vi "RAMP SPEED.vi"(8 "error in (no error)":errorcluster, 11 "main ref":T1) -> (0 "error out":errorcluster)   [LabVIEW 2025]
uses:
  controls/LAB-IQ UI Data.ctl
  SWAY vi's/Sway Write enum.ctl
  <vilib>/Analysis/1siggen.llb/Ramp Pattern by Samples.vi
  <vilib>/Analysis/NI_AALBase.lvlib
  HEAVE vi's/Heave Write enum.ctl
panel:
  out "Initial Rpm":dbl
  out "Wait Time":dbl
  out "Total Steps":dbl
  out "Speed":dbl
  out "Ramp Pattern":dbl[](array[numeric])
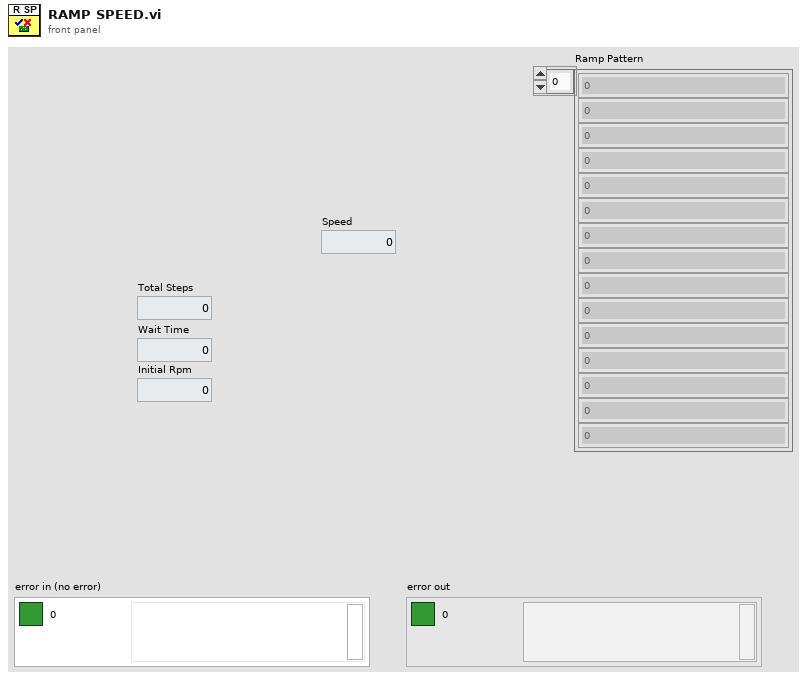
[diagram p1: front panel]
types:
  T1 = typedef "LAB-IQ UI Data.ctl" = cluster{"Main Home Screen":cluster{"GUI":refnum<vi>, "Platform Settings":refnum<vi>, "Configure":refnum<vi>, "Home":refnum<vi>, "EXIT":refnum<vi>, "service 2":refnum<vi>, "MainPage":refnum<vi>, "Analysis":refnum<vi>}, "Platform Settings":cluster{"mm/s  Surge":refnum<vi>, "Update Surge Speed":refnum<vi>, "Drive Error":refnum<vi>, "Disable Axis Jog Soft Limits":refnum<vi>, "mm/s  Sway":refnum<vi>, "Sway and Surge COM Status":refnum<vi>, "Heave COM Status":refnum<vi>, "Enable Platform":refnum<vi>, "Surge Forward Main":refnum<vi>, "Sway Right Main":refnum<vi>, "Sway Left Main":refnum<vi>, "Heave Down Main":refnum<vi>, "Heave Up main":refnum<vi>, "Update Sway Speed":refnum<vi>, "Update Heave Speed":refnum<vi>, "mm/s Heave":refnum<vi>, "mm/sec":refnum<vi>, "mm":refnum<vi>, "Surge Backward Main":refnum<vi>}, "Analysis Screen":cluster{"Analysis Home":refnum<vi>, "Surface Analysis":refnum<vi>, "Imaging":refnum<vi>, "Image Analysis":refnum<vi>, "Post Analysis":refnum<vi>}, "Config Screen":cluster{"Select Load Head":refnum<vi>, "Notes :":refnum<vi>, "FILE":refnum<vi>, "Sample ID :":refnum<vi>, "Operator ID :":refnum<vi>, "Operator Name :":refnum<vi>, "Auto":refnum<vi>}, "Motion Module":cluster{"zNL":refnum<vi>, "NL disp":refnum<vi>, "Rotary Tab":refnum<vi>, "Motion Direction:  3":refnum<vi>, "E.Velocity 2":refnum<vi>, "e.v/ssr 2":refnum<vi>, "Enter Fixed E.Velocity 2":refnum<vi>, "Enter Final SRR 2":refnum<vi>, "Enter initial SRR 2":refnum<vi>, "Enter Fixed SRR 2":refnum<vi>, "Enter the Final E.Velocity (m/s) 2":refnum<vi>, "Enter initial E.Velocity (m/s) 2":refnum<vi>, "Final Speed (RPM) 3":refnum<vi>, "Initial Speed (RPM) 2":refnum<vi>, "Enter the Final Velocity (m/s) 3":refnum<vi>, "Enter initial Velocity (m/s)  3":refnum<vi>, "Ramp Up 2":refnum<vi>, "TEST SELECTION":refnum<vi>, "SPEED SELECTION : ":refnum<vi>, "Angular Oscillation Set":refnum<vi>, "Traction":refnum<vi>, "Step Speed":refnum<vi>, "StepTable For Load-Speed":refnum<vi>, "StepTable For Speed":refnum<vi>, "Surge Forward MM":refnum<vi>, "Surge Backward MM":refnum<vi>, "M3 Image":refnum<vi>, "String 39":refnum<vi>, "Sway Left MM":refnum<vi>, "Sway Right MM":refnum<vi>, "Disable Axis Jog Soft Limits":refnum<vi>, "mm":refnum<vi>, "Heave Down MM":refnum<vi>, "Heave Up MM":refnum<vi>, "Wear Track Diameter (mm)":refnum<vi>, "Set WTD":refnum<vi>, "HomeScratch":refnum<vi>, "HomeRot":refnum<vi>, "PlaceModule":refnum<vi>, "Enter the Angle (Deg)":refnum<vi>, "Enter the Frequency (Hz)":refnum<vi>, "Motion Mode:":refnum<vi>, "LR Sway":refnum<vi>, "Rot Hor":refnum<vi>, "Scratch":refnum<vi>, "LR Cam":refnum<vi>, "MMBack":refnum<vi>, "MMNext":refnum<vi>, "Rot Ver":refnum<vi>, "Rotary Module Selection":refnum<vi>, "calculate rotary":refnum<vi>, "SPEED SELECTION : rotary":refnum<vi>, "Import 2":refnum<vi>, "Save 2":refnum<vi>, "File Path :  2":refnum<vi>, "String 45":refnum<vi>, "StepTable For Speed 3":refnum<vi>, "Enter the Speed(mm/sec)":refnum<vi>, "Enter the Speed(RPM)":refnum<vi>, "Enter Scratch Speed (mm/s):":refnum<vi>, "SwaySpeed Set":refnum<vi>, "Scartch Offset":refnum<vi>, "Motion type:":refnum<vi>, "HomeScratch 2":refnum<vi>, "Enter Scratch length (mm):":refnum<vi>, "Wear Track Diameter":refnum<vi>, "Rotary Speed Exced":refnum<vi>, "Scratch Mode":refnum<vi>, "No of Scratch":refnum<vi>}, "Environmental control":cluster{"Humidity  Status  3":refnum<vi>, "Low Temp  Status  2":refnum<vi>, "TK4 status 2":refnum<vi>, "Stage Temperature":refnum<vi>, "Sample Temperature":refnum<vi>, "Humidity (Amb)":refnum<vi>, "Clear List":refnum<vi>, "Add to list":refnum<vi>, "Wear":refnum<vi>, "Vibration":refnum<vi>, "Humidity (Chamber)":refnum<vi>, "Temperature (Chamber)":refnum<vi>, "ECR ":refnum<vi>, "Temperature (Amb)":refnum<vi>, "Microphone":refnum<vi>, "Acoustic Emission 3":refnum<vi>, "SNext":refnum<vi>, "APBack":refnum<vi>, "Enter the Temperature (°C):":refnum<vi>, "Enter the Stage \nTemperature (°C):":refnum<vi>, "Enter the Humidity (%Rh):":refnum<vi>, "Low Temp":refnum<vi>, "High Temp":refnum<vi>, "Humidity":refnum<vi>, "Sensors Picked":refnum<vi>}, "About Screen":cluster{"Password":refnum<vi>, "Home Service":refnum<vi>, "Advanced Setting":refnum<vi>, "About Tab":refnum<vi>, "ECR Port:":refnum<vi>, "Ramp Port:":refnum<vi>, "Installation/Replacement completed":refnum<vi>, "Loahead":refnum<vi>, "Heave and Surge COM Port:":refnum<vi>, "Sway COM Port:":refnum<vi>, "Temp Modbus:":refnum<vi>, "Humidity Port:":refnum<vi>, "Edit Gain Constants":refnum<vi>, "Save Gain Constants":refnum<vi>}, "Main Screen":cluster{"Main Screen Tab":refnum<vi>, "Angle and Frequency":refnum<vi>, "Stroke (mm)":refnum<vi>, "Angle (Deg)":refnum<vi>, "Main Speed Tab":refnum<vi>, "MTM MOTOR DISPLAY":refnum<vi>, "Disc Speed (m/sec)":refnum<vi>, "Ball Speed (m/sec)":refnum<vi>, "Disc Speed (RPM)":refnum<vi>, "Ball Speed (RPM)":refnum<vi>, "SPEED TAB":refnum<vi>, "Speed (m/sec)":refnum<vi>, "Set Speed (m/sec)":refnum<vi>, "Speed (RPM)":refnum<vi>, "Set Speed":refnum<vi>, "Time Tab":refnum<vi>, "Time ( HH:MM:SS ) 2":refnum<vi>, "Test Duration":refnum<vi>, "Test Duration 4":refnum<vi>, "TEST CYCLE":refnum<vi>, "TOTAL CYCLES":refnum<vi>, "Set Load (N)":refnum<vi>, "Temp Tabs":refnum<vi>, "Heater":refnum<vi>, "TK4 status":refnum<vi>, "ChamberTemp":refnum<vi>, "SetTmp":refnum<vi>, "Controller  Status":refnum<vi>, "ChamberTemp 2":refnum<vi>, "SetTmp 2":refnum<vi>, "Controller  Status 2":refnum<vi>, "ChamberTemp 3":refnum<vi>, "SetTmp 3":refnum<vi>, "Cooling":refnum<vi>, "Load Communication":refnum<vi>, "Ambient \nTemperature":refnum<vi>, "HumCOMStatus":refnum<vi>, "Ambient\n Humidity":refnum<vi>, "Freq (Hz)":refnum<vi>, "Load En":refnum<vi>, "NLt":refnum<vi>, "zNL 2":refnum<vi>, "Humidity On":refnum<vi>, "humidity disp":refnum<vi>, "Set Humidity":refnum<vi>, "NL disp 2":refnum<vi>, "Humidity On 2":refnum<vi>, "humidity disp 2":refnum<vi>, "Set Humidity 2":refnum<vi>, "NL disp 3":refnum<vi>, "AppLoadSeq scratch":refnum<vi>, "Stop Scratch":refnum<vi>, "ClrLog":refnum<vi>, "Trip Log":refnum<vi>, "STOP":refnum<vi>, "Start Test":refnum<vi>, "Test status":refnum<vi>, "AR Led":refnum<vi>, "Data":refnum<vi>, "Health":refnum<vi>, "Sway COM Status":refnum<vi>, "Heave COM Status":refnum<vi>, "Grp Tab":refnum<vi>, "Sub Graph":refnum<vi>, "SD (mm)":refnum<vi>, "Siliding distance Reset Graph":refnum<vi>, "SDGp":refnum<vi>, "Humidity Reset Graph":refnum<vi>, "HumrGp":refnum<vi>, "Acoustic Emission (mV)":refnum<vi>, "Aqucostic Reset Graph":refnum<vi>, "gACQUOS":refnum<vi>, "ECR RESET":refnum<vi>, "ECR":refnum<vi>, "Temperature Reset":refnum<vi>, "Acoustic Emission (mV) 2":refnum<vi>, "Aqucostic Reset Graph 2":refnum<vi>, "gACQUOS 2":refnum<vi>, "ECR RESET 2":refnum<vi>, "ECR 2":refnum<vi>, "Temperature Reset 2":refnum<vi>, "Temperature (deg c)":refnum<vi>, "Speed Reset Graph":refnum<vi>, "Speed Tab":refnum<vi>, "MTM DISC  SPEED":refnum<vi>, "MTM BALL SPEED":refnum<vi>, "speed mm/sec":refnum<vi>, "Hymidity":refnum<vi>, "Humidity Disable trip":refnum<vi>, "CoF Trip  2":refnum<vi>, "Depth Trip":refnum<vi>, "Weart Deapth":refnum<vi>, "Depth Reset Graph":refnum<vi>, "Weart":refnum<vi>, "Depthz":refnum<vi>, "Depth (µm)":refnum<vi>, "WearGp":refnum<vi>, "NL Trip 2":refnum<vi>, "Load pid":refnum<vi>, "Load Disable Trip":refnum<vi>, "Load Reset Graph":refnum<vi>, "NL Display 4":refnum<vi>, "Main Chart 3":refnum<vi>, "BACK":refnum<vi>, "Depth Trip 2":refnum<vi>, "COF TRIP ":refnum<vi>, "Friction Force (N)":refnum<vi>, "FF Reset Graph":refnum<vi>, "FF Disable Trip":refnum<vi>, "FF TRIP":refnum<vi>, "COF Disable Trip":refnum<vi>, "COF Reset Graph":refnum<vi>, "Start Test Temp":refnum<vi>, "zFF":refnum<vi>, "Friction Force (N) Graph":refnum<vi>, "Coefficient of Friction":refnum<vi>, "Scratch Start Test":refnum<vi>, "FF Tab":refnum<vi>, "Cyclic Friction Force (N)":refnum<vi>, "CZ FF":refnum<vi>, "Cyclic Friction Force (N) Graph":refnum<vi>, "Cyclic Coefficient of Friction":refnum<vi>, "Cyclic FF TRIP":refnum<vi>, "Cyclic FF Disable Trip":refnum<vi>, "cyclic COF Disable Trip":refnum<vi>, "cyclic COF TRIP":refnum<vi>, "cyclic COF Reset Graph":refnum<vi>, "Cyclic FF Reset Graph":refnum<vi>, "Test Trip":refnum<vi>, "Multi Scratch Pass":refnum<vi>, "Scratch Start Recording":refnum<vi>}, "Loading":cluster{"Indentation":refnum<vi>, "Reference Sample":refnum<vi>, "Load Cell Communication Slide":refnum<vi>, "com 3":refnum<vi>, "com":refnum<vi>, "DecaForce COM Status":refnum<vi>, "Update":refnum<vi>, "Clear 3":refnum<vi>, "seq":refnum<vi>, "Stribeck table":refnum<vi>, "Stribeck Table  For loading":refnum<vi>, "Loading Mode":refnum<vi>, "Enter the Final Load (N)":refnum<vi>, "Enter the CoF Trip":refnum<vi>, "Enter the Friction Force Trip":refnum<vi>, "Enter the Normal load Trip":refnum<vi>, "Enter the Load  (N)":refnum<vi>, "KiloForce":refnum<vi>, "DecaForce ":refnum<vi>, "MicroForce":refnum<vi>, "LHBack":refnum<vi>, "LHNext":refnum<vi>, "Enter the Loading Rate (N/min)":refnum<vi>, "Message":refnum<vi>, "Warning 2":refnum<vi>, "SSP 0.75":refnum<vi>, "SSP 0.5":refnum<vi>, "SSP 0.3":refnum<vi>, "Warning":refnum<vi>, "gui GIF":refnum<vi>, "Communication is established":refnum<vi>, "AppLoad 4":refnum<vi>, "Multipoint":refnum<vi>, "Load Selection":refnum<vi>}, "PID":cluster{"Ramp MulFac":refnum<vi>, "pulses LoadDiffRamp(2..10)":refnum<vi>, "PulseControlRamp(diff<=3N)":refnum<vi>, "SetLoadDeadband(%) Load(0-10N)":refnum<vi>, "PID gains out delay (microForce)":refnum<vi>, "Ramp":refnum<vi>, "Gain 2":refnum<vi>, "pulses LoadDiff(2..10)":refnum<vi>, "pulses LoadDiff(11..50)":refnum<vi>, "PulseControl(diff<=3N)":refnum<vi>, "SetLoadDeadband(%)  2":refnum<vi>, "Dummy Run":refnum<vi>, "Vertical load (N)":refnum<vi>, "AutoTune":refnum<vi>, "Offset 3 ":refnum<vi>, "apply load":refnum<vi>, "Offset  3":refnum<vi>, "apply load 2":refnum<vi>, "Enter ByPass Load":refnum<vi>, "reinit 3":refnum<vi>, "output range delay":refnum<vi>, "PID gains out delay":refnum<vi>, "Bypass Load":refnum<vi>, "pulsesSent":refnum<vi>, "pulses ":refnum<vi>, "actpid":refnum<vi>, "gFF Rot":refnum<vi>, "pulses LoadDiff(21..1000)":refnum<vi>, "Delay":refnum<vi>, "deadband":refnum<vi>}, "Config Parameters":cluster{"Tab Control 3":refnum<vi>, "Tab Control 19":refnum<vi>, "SAMPLES":refnum<vi>, "Re-initilaize":refnum<vi>, "Filter ON/OFF":refnum<vi>, "TracHomeSurgeOffsetCounts 10MM":refnum<vi>, "TracHomeSwayOffsetCounts 10MM":refnum<vi>, "Acoustic Emission:":refnum<vi>, "Apply Filter (FF)":refnum<vi>, "Filter% 2":refnum<vi>, "Apply Filter (Load)":refnum<vi>, "Filter% ":refnum<vi>, "Sway distance (mm)":refnum<vi>, "Surge distance (mm)":refnum<vi>, "DataSavingLoopDelay(ms)":refnum<vi>, "SAVE 2":refnum<vi>, "Enter Distance":refnum<vi>, "Sway Counts:":refnum<vi>, "Distance (mm): 3":refnum<vi>, "Surge Counts:":refnum<vi>, "Distance (mm): 2":refnum<vi>, "Distance (mm):":refnum<vi>, "Heave Counts:":refnum<vi>, "LRMHomeSurgeOffsetCounts":refnum<vi>, "LRMHomeSwayOffsetCounts":refnum<vi>, "TracHomeSurgeOffsetCounts 20MM":refnum<vi>, "TracHomeSwayOffsetCounts 20MM":refnum<vi>, "RotHomeSwayOffsetCounts":refnum<vi>, "RotHomeSurgeOffsetCounts":refnum<vi>, "Heave distance":refnum<vi>, "Zmm":refnum<vi>, "Heave Pulses/mm":refnum<vi>, "Surge Pulses/mm":refnum<vi>, "Sway Pulses/mm":refnum<vi>, "Heave Pitch":refnum<vi>, "Surge Pitch":refnum<vi>, "Sway Pitch":refnum<vi>, "Heave PPR":refnum<vi>, "Surge PPR":refnum<vi>, "Sway PPR":refnum<vi>, "Tab Control 5":refnum<vi>, "Tab Control 14":refnum<vi>, "Tab Control 26":refnum<vi>, "AE":refnum<vi>, "Heave Loop Delay":refnum<vi>, "Heave PID Speed":refnum<vi>, "Surge Jog Speed":refnum<vi>, "Heave Jog Speed":refnum<vi>, "Sway Loop Delay":refnum<vi>, "Sway PID Speed":refnum<vi>, "Sway Jog Speed":refnum<vi>, "DEPTH TRIP VALUE":refnum<vi>, "LOAD TRIP VALUE":refnum<vi>, "DEPTH TRIP   ENABLE":refnum<vi>, "LOAD TRIP  ENABLE":refnum<vi>, "CYCLIC FF TRIP VALUE":refnum<vi>, "FF TRIP VALUE":refnum<vi>, "CYCLIC CoF TRIP VALUE":refnum<vi>, "COF TRIP VALUE":refnum<vi>, "CYCLIC COF TRIP  ENABLE":refnum<vi>, "CYCLIC FF TRIP  ENABLE":refnum<vi>, "FF TRIP  ENABLE":refnum<vi>, "COF TRIP  ENABLE":refnum<vi>}, "Loading Com Port":cluster{"ClearAll":refnum<vi>, "Mz(Nm)":refnum<vi>, "My(Nm)":refnum<vi>, "Mx(Nm)":refnum<vi>, "Save Dwell":refnum<vi>, "Mx ":refnum<vi>, "My ":refnum<vi>, "Mz":refnum<vi>, "Fx(N)":refnum<vi>, "Fy(N)":refnum<vi>, "Fz(N)":refnum<vi>, "ZeroAll":refnum<vi>, "Acq Delay (ms)":refnum<vi>, "Burst Delay (ms)":refnum<vi>, "model":refnum<vi>, "SN":refnum<vi>, "FFx(N)":refnum<vi>, "Sensor IP":refnum<vi>, "Port":refnum<vi>, "FFy(N)":refnum<vi>, "Load(N)":refnum<vi>, "delete Handle":refnum<vi>, "Create Handle":refnum<vi>, "ft_data":refnum<vi>, "ft_range":refnum<vi>, "ft_data 2":refnum<vi>, "stop 6":refnum<vi>, "running_flag":refnum<vi>, "ft_udp_handle":refnum<vi>, "get-data-return":refnum<vi>, "get-range-return":refnum<vi>, "zero-return":refnum<vi>, "filter-return":refnum<vi>, "initial-return":refnum<vi>, "deleteHandle-result":refnum<vi>, "Load Cell Temp":refnum<vi>}, "Heave AND Surge":cluster{"SURGE POSE":refnum<vi>, "error out Read":refnum<vi>, "HEAVE POSE":refnum<vi>, "State":refnum<vi>, "Homed":refnum<vi>, "Sequence ID":refnum<vi>, "error out Write":refnum<vi>, "faultCode":refnum<vi>, "Ack ID":refnum<vi>, "SPEED":refnum<vi>, "Distance":refnum<vi>, "Mode Command":refnum<vi>, "Heave and Surge Read":refnum<vi>, "Read Heave Temp":refnum<vi>, "Spare 15":refnum<vi>, "Spare 14":refnum<vi>, "Spare 13":refnum<vi>, "Spare 12":refnum<vi>, "Spare 11":refnum<vi>, "Spare 10":refnum<vi>, "Spare 9":refnum<vi>, "Spare 8":refnum<vi>, "Spare 7":refnum<vi>, "Spare 6":refnum<vi>, "Spare 5":refnum<vi>, "Spare 4":refnum<vi>, "Spare 2":refnum<vi>, "Spare 1":refnum<vi>, "Node Id":refnum<vi>, "Spare 3":refnum<vi>, "SPARE 4":refnum<vi>, "SPARE 3":refnum<vi>, "SPARE 2":refnum<vi>, "SPARE 1":refnum<vi>, "fwMajor":refnum<vi>, "fwMinor":refnum<vi>, "Manual Write":refnum<vi>, "Heave and Surge Write":refnum<vi>}, "New PID LOGIC":cluster{"Fine Tune Zone":refnum<vi>, "PID SDelay":refnum<vi>, "Max_pos_limit":refnum<vi>, "Min_pos_limit":refnum<vi>, "i_limit":refnum<vi>, "pct_scale":refnum<vi>, "Deadband":refnum<vi>, "Kd":refnum<vi>, "Ki":refnum<vi>, "Kp":refnum<vi>, "Current Position":refnum<vi>, "Set Load":refnum<vi>, "Current Load":refnum<vi>, "Pulse delta":refnum<vi>, "Init Step":refnum<vi>, "Max Step Linit":refnum<vi>}, "SWAY ":cluster{"fwMajor":refnum<vi>, "Homed":refnum<vi>, "Rotary POSE":refnum<vi>, "State":refnum<vi>, "SWAY POSE":refnum<vi>, "Ack ID":refnum<vi>, "faultCode":refnum<vi>, "Node Id":refnum<vi>, "fwMinor":refnum<vi>, "Spare 6":refnum<vi>, "Spare 5":refnum<vi>, "Spare 4":refnum<vi>, "Spare 3":refnum<vi>, "Spare 2":refnum<vi>, "Spare 1":refnum<vi>, "Spare 7":refnum<vi>, "SPARE  5":refnum<vi>, "error out Write  SWAY ":refnum<vi>, "error out Read SWAY ":refnum<vi>, "Manual Write SWAY ":refnum<vi>, "SWAY WRITE":refnum<vi>, "SPARE  4":refnum<vi>, "SPARE  3":refnum<vi>, "SPARE 2":refnum<vi>, "SPARE 1":refnum<vi>, "Spare 15":refnum<vi>, "Spare 14":refnum<vi>, "Spare 13":refnum<vi>, "Spare 12":refnum<vi>, "Spare 11":refnum<vi>, "Spare 9":refnum<vi>, "Spare 8":refnum<vi>, "SPEED":refnum<vi>, "Distance":refnum<vi>, "Mode Command":refnum<vi>, "Sequence ID":refnum<vi>, "SWAY READ":refnum<vi>, "Spare 10":refnum<vi>, "Read SWAY Temp":refnum<vi>}, "Analysis Screen":cluster{"Analysis Home":refnum<vi>, "Refresh 2":refnum<vi>, "MEAN 4":refnum<vi>, "SD 4":refnum<vi>, "VARIANCE 4":refnum<vi>, "MEAN  3":refnum<vi>, "SD  3":refnum<vi>, "VARIANCE  3":refnum<vi>, "MEAN 2":refnum<vi>, "SD  2":refnum<vi>, "VARIANCE 2":refnum<vi>, "MEAN":refnum<vi>, "SD":refnum<vi>, "VARIANCE":refnum<vi>, "File 4 Discription":refnum<vi>, "OPEN 4":refnum<vi>, "File Name 4":refnum<vi>, "OPEN 3":refnum<vi>, "File 3 Discription":refnum<vi>, "File Name 3":refnum<vi>, "Y-AXIS":refnum<vi>, "X-AXIS":refnum<vi>, "XY Graph":refnum<vi>, "File Name 2":refnum<vi>, "File Name 1":refnum<vi>, "OPEN 2":refnum<vi>, "OPEN 1":refnum<vi>, "File 1 Discription ":refnum<vi>, "File 2 Discription":refnum<vi>, "Export":refnum<vi>, "File Format":refnum<vi>}}
  T2 = enum32{"Setup", "Load Head", "Motion Module", "Environment", "Begin"}
  T3 = typedef "Sway Write enum.ctl" = enum16{"INIT", "WRITE", "CLOSE", "REINIT"}
  T4 = typedef "Heave Write enum.ctl" = enum16{"INIT", "WRITE", "CLOSE", "REINIT"}
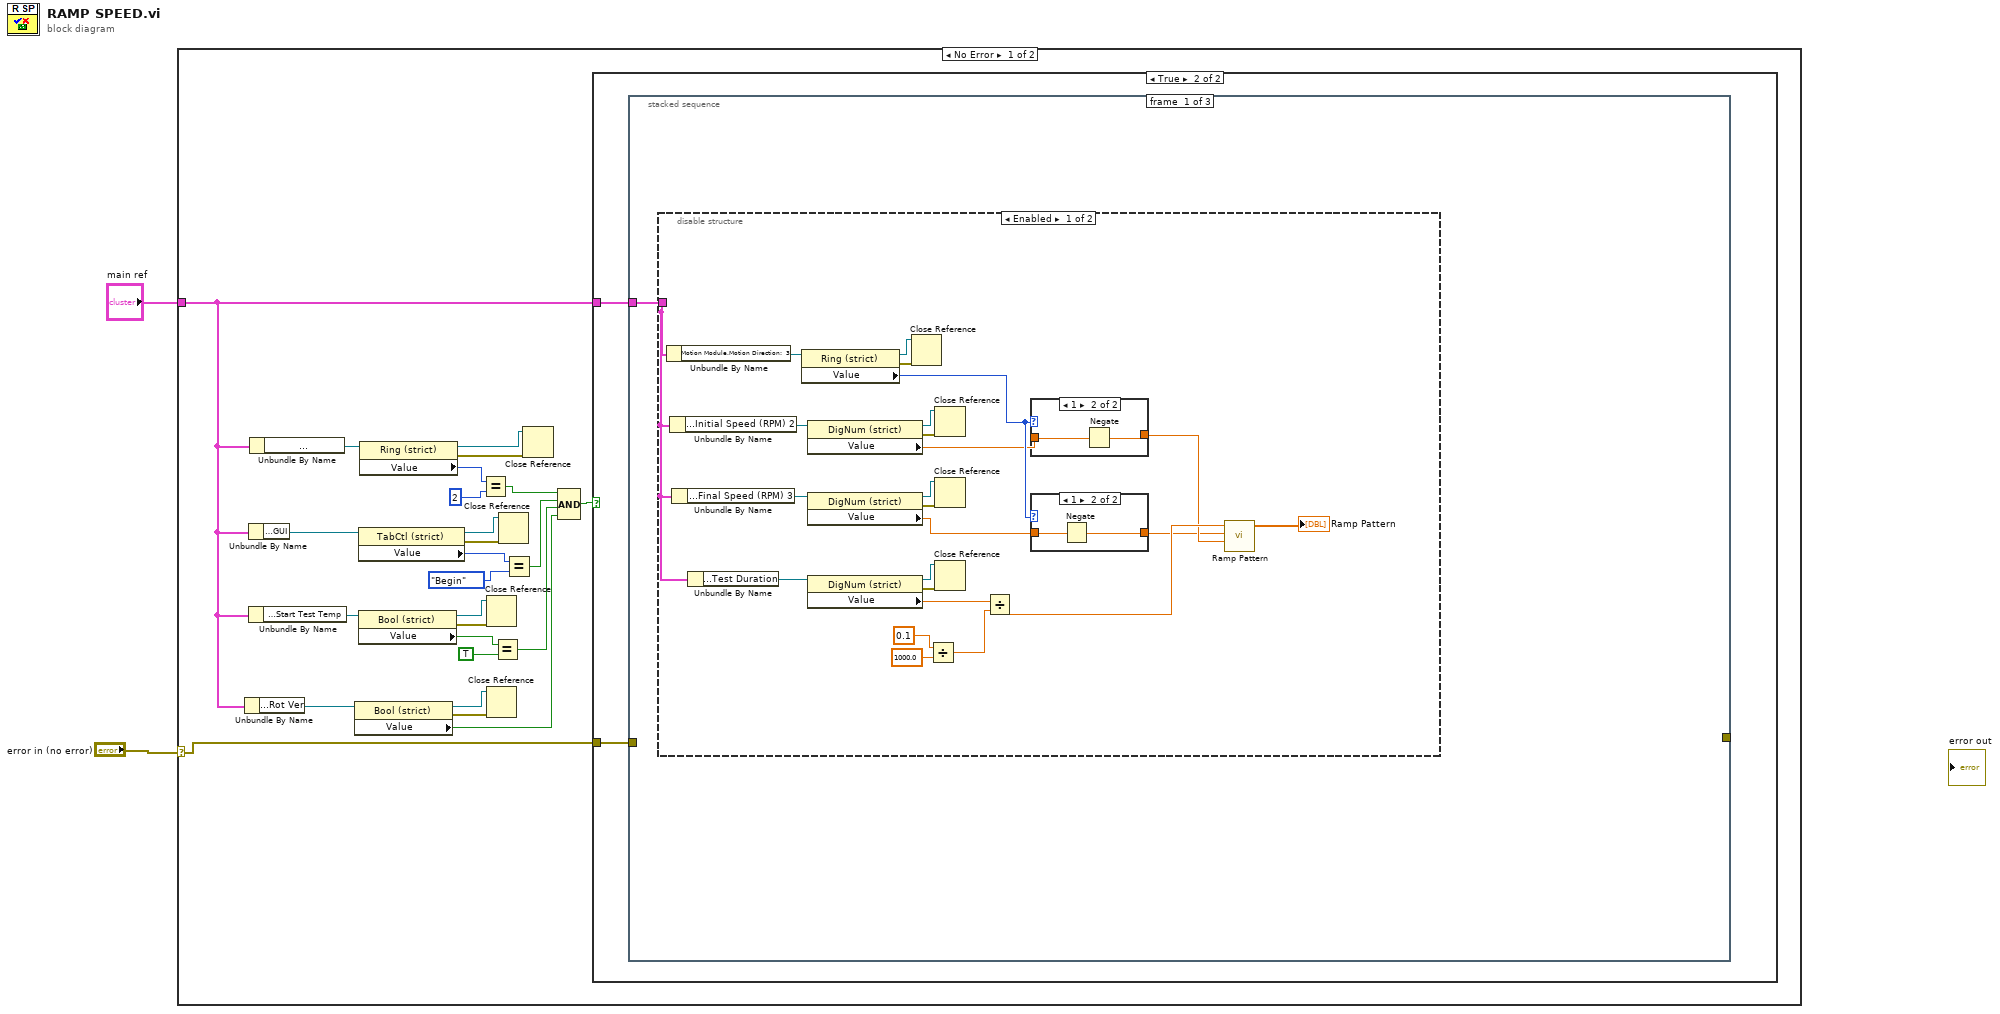
[diagram p0: block diagram]
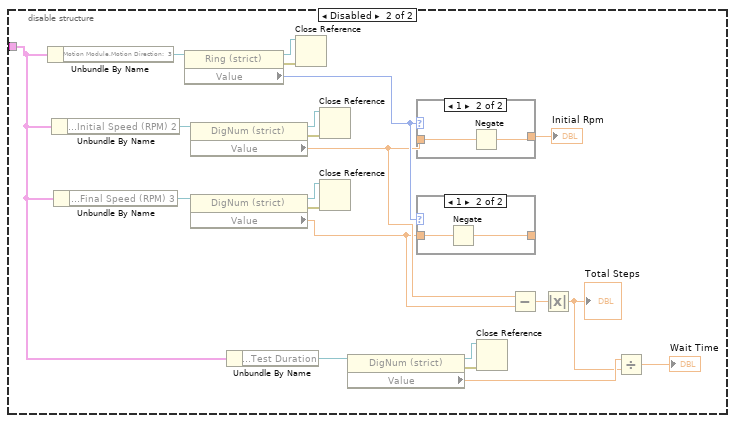
[diagram p5: hidden frame]
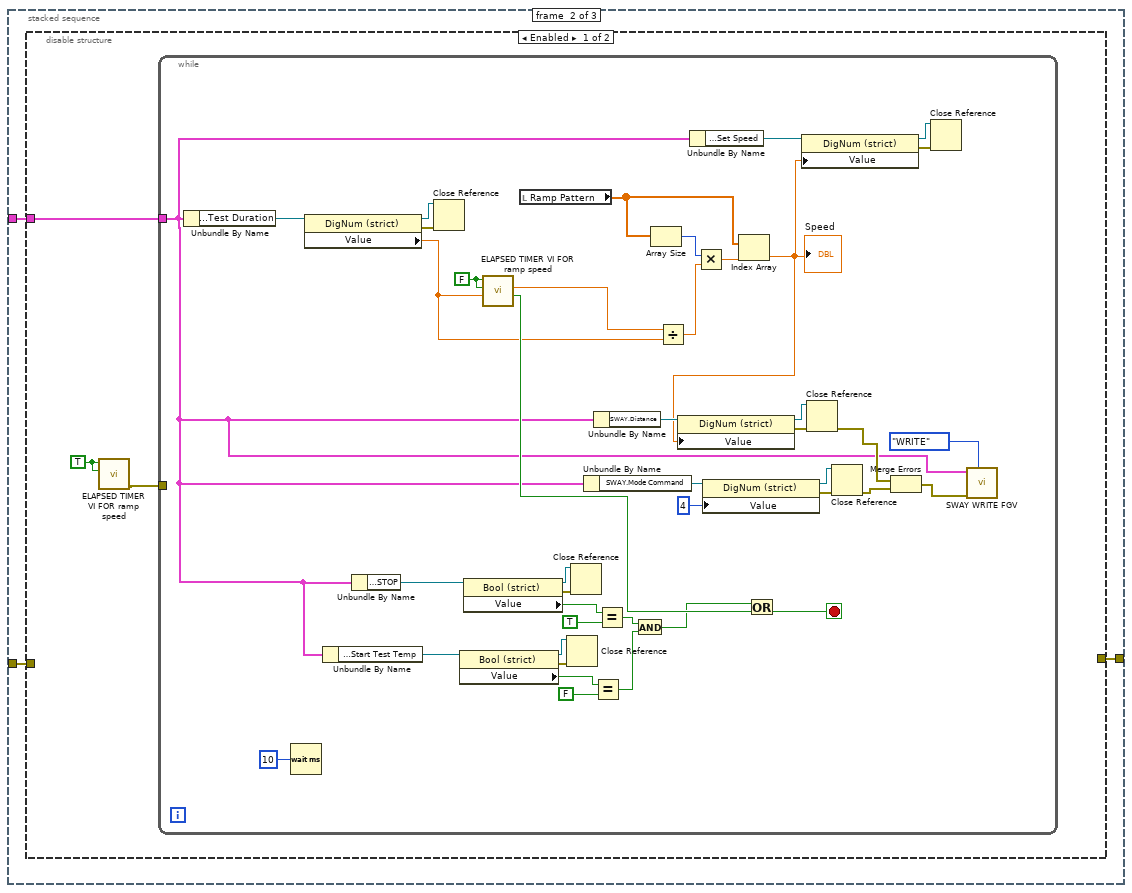
[diagram p8: hidden frame]
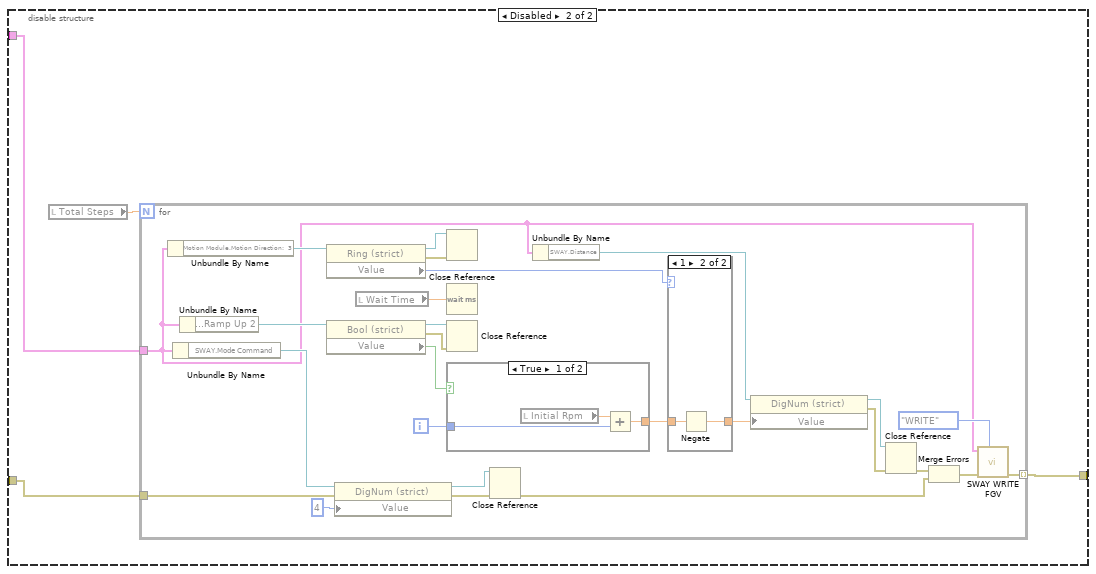
[diagram p9: hidden frame]
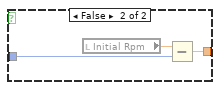
[diagram p10: hidden frame]
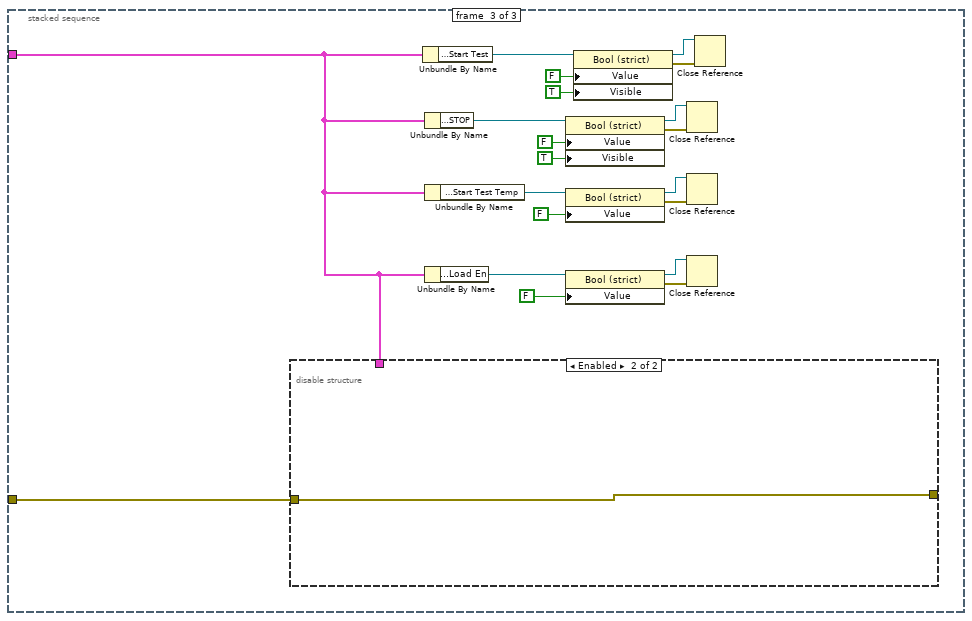
[diagram p12: hidden frame]
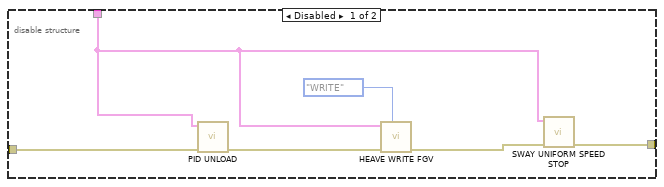
[diagram p13: hidden frame]
diagram:
  n1 = case shown="No Error" "error in (no error)" {
    selector: "error in (no error)" -> [w3 _]
    tunnel: "main ref" -> [w5 _]
    frame No Error {
      n2 = Unbundle By Name(w5) -> ("Motion Module.Rot Ver"=w9:refnum<vi>)
      n3 = Unbundle By Name(w5) -> ("Main Home Screen.GUI"=w19:refnum<vi>)
      n4 = Unbundle By Name(w5) -> ("Main Screen.Start Test Temp"=w14:refnum<vi>)
      n5 = Unbundle By Name(w5) -> ("Motion Module.Motion Mode:"=w27:refnum<vi>)
      n6 = property class="Bool (strict)"(reference=w9) -> (reference out=w6:refnum<vi>, error out=w8:errorcluster, "Value"=w7:bool)  [unwired: 1 in]
      n7 = property class="TabCtl (strict)"(reference=w19) -> (reference out=w21:refnum<vi>, error out=w20:errorcluster, "Value"=w18:T2)  [unwired: 1 in]
      n8 = property class="Bool (strict)"(reference=w14) -> (reference out=w12:refnum<vi>, error out=w13:errorcluster, "Value"=w15:bool)  [unwired: 1 in]
      n9 = property class="Ring (strict)"(reference=w27) -> (reference out=w25:refnum<vi>, error out=w26:errorcluster, "Value"=w24:u16)  [unwired: 1 in]
      n10 = Equal?(x=w24, y=u16 2 ("Value")) -> (x = y?=w22:bool)
      n11 = Close Reference(reference=w12, error in (no error)=w13) -> ()  [unwired: 1 out]
      n12 = Close Reference(reference=w6, error in (no error)=w8) -> ()  [unwired: 1 out]
      n13 = Equal?(x=w15, y=TRUE) -> (x = y?=w11:bool)
      n14 = Close Reference(reference=w21, error in (no error)=w20) -> ()  [unwired: 1 out]
      n15 = Equal?(x=w18, y=T2."Begin" ("Value")) -> (x = y?=w16:bool)
      n16 = Close Reference(reference=w25, error in (no error)=w26) -> ()  [unwired: 1 out]
      n17 = Compound Arithmetic op=AND(w22, w16, w11, w7) -> (w4:bool)
      n18 = case shown="True" w4 {
        tunnel: w5 -> [_ w29]
        tunnel: w3 -> [_ w28]
        frame False {
        }
        frame True {
          n19 = stacked-sequence {
            tunnel: w29 -> [w30 w90 w175]
            tunnel: w28 -> [_ w89 w176]
            tunnel: [_ w88 _] -> _
            frame #0 {
              n20 = disable-structure shown="Enabled" {
                disable-tunnel: w30 -> [w32 w68]
                frame Enabled {
                  n21 = Unbundle By Name(w32) -> ("Motion Module.Motion Direction:  3"=w47:refnum<vi>)
                  n22 = Unbundle By Name(w32) -> ("Motion Module.Initial Speed (RPM) 2"=w41:refnum<vi>)
                  n23 = Unbundle By Name(w32) -> ("Motion Module.Final Speed (RPM) 3"=w40:refnum<vi>)
                  n24 = Unbundle By Name(w32) -> ("Main Screen.Test Duration"=w33:refnum<vi>)
                  n25 = property class="Ring (strict)"(reference=w47) -> (reference out=w45:refnum<vi>, error out=w46:errorcluster, "Value"=w44:u16)  [unwired: 1 in]
                  n26 = property class="DigNum (strict)"(reference=w41) -> (reference out=w43:refnum<vi>, error out=w42:errorcluster, "Value"=w36:dbl)  [unwired: 1 in]
                  n27 = property class="DigNum (strict)"(reference=w40) -> (reference out=w38:refnum<vi>, error out=w39:errorcluster, "Value"=w37:dbl)  [unwired: 1 in]
                  n28 = property class="DigNum (strict)"(reference=w33) -> (reference out=w35:refnum<vi>, error out=w34:errorcluster, "Value"=w31:dbl)  [unwired: 1 in]
                  n29 = Close Reference(reference=w45, error in (no error)=w46) -> ()  [unwired: 1 out]
                  n30 = Divide(x=0.1 ("seconds to wait"), y=1000.0) -> (x/y=w54:dbl)
                  n31 = Close Reference(reference=w43, error in (no error)=w42) -> ()  [unwired: 1 out]
                  n32 = Close Reference(reference=w38, error in (no error)=w39) -> ()  [unwired: 1 out]
                  n33 = Close Reference(reference=w35, error in (no error)=w34) -> ()  [unwired: 1 out]
                  n34 = Divide(x=w31, y=w54) -> (x/y=w53:dbl)
                  n35 = case shown="1" w44 {
                    tunnel: w36 -> [w58 w60]
                    tunnel: [w58 w59] -> w52
                    frame 0, Default {
                    }
                    frame 1 {
                      n36 = Negate(x=w60) -> (-x=w59:dbl)
                    }
                  }
                  n37 = case shown="1" w44 {
                    tunnel: w37 -> [w55 w57]
                    tunnel: [w55 w56] -> w51
                    frame 0, Default {
                    }
                    frame 1 {
                      n38 = Negate(x=w57) -> (-x=w56:dbl)
                    }
                  }
                  n39 = call-poly <vilib>:"Ramp Pattern.vi"("start"=w52, "end"=w51, "samples"=w53) -> ("Ramp Pattern"=→"Ramp Pattern":dbl[])  [unwired: 7 in, 1 out]
                }
                frame Disabled {
                  n40 = Unbundle By Name(w68) -> ("Motion Module.Motion Direction:  3"=w81:refnum<vi>)
                  n41 = Unbundle By Name(w68) -> ("Motion Module.Initial Speed (RPM) 2"=w75:refnum<vi>)
                  n42 = Unbundle By Name(w68) -> ("Motion Module.Final Speed (RPM) 3"=w74:refnum<vi>)
                  n43 = property class="Ring (strict)"(reference=w81) -> (reference out=w79:refnum<vi>, error out=w80:errorcluster, "Value"=w78:u16)  [unwired: 1 in]
                  n44 = property class="DigNum (strict)"(reference=w75) -> (reference out=w77:refnum<vi>, error out=w76:errorcluster, "Value"=w67:dbl)  [unwired: 1 in]
                  n45 = property class="DigNum (strict)"(reference=w74) -> (reference out=w72:refnum<vi>, error out=w73:errorcluster, "Value"=w66:dbl)  [unwired: 1 in]
                  n46 = Unbundle By Name(w68) -> ("Main Screen.Test Duration"=w69:refnum<vi>)
                  n47 = Close Reference(reference=w79, error in (no error)=w80) -> ()  [unwired: 1 out]
                  n48 = Close Reference(reference=w77, error in (no error)=w76) -> ()  [unwired: 1 out]
                  n49 = Close Reference(reference=w72, error in (no error)=w73) -> ()  [unwired: 1 out]
                  n50 = property class="DigNum (strict)"(reference=w69) -> (reference out=w71:refnum<vi>, error out=w70:errorcluster, "Value"=w65:dbl)  [unwired: 1 in]
                  n51 = case shown="1" w78 {
                    tunnel: w67 -> [w85 w87]
                    tunnel: [w85 w86] -> w61
                    frame 0, Default {
                    }
                    frame 1 {
                      n52 = Negate(x=w87) -> (-x=w86:dbl)
                    }
                  }
                  "Initial Rpm" <- w61
                  n53 = case shown="1" w78 {
                    tunnel: w66 -> [w82 w84]
                    tunnel: [w82 w83] -> _
                    frame 0, Default {
                    }
                    frame 1 {
                      n54 = Negate(x=w84) -> (-x=w83:dbl)
                    }
                  }
                  n55 = Close Reference(reference=w71, error in (no error)=w70) -> ()  [unwired: 1 out]
                  n56 = Subtract(x=w67, y=w66) -> (x-y=w64:dbl)
                  n57 = Absolute Value(x=w64) -> (abs(x)=w63:dbl)
                  "Total Steps" <- w63
                  n58 = Divide(x=w65, y=w63) -> (x/y=→"Wait Time":dbl)
                }
              }
            }
            frame #1 {
              n59 = disable-structure shown="Enabled" {
                disable-tunnel: w90 -> [w91 w138]
                disable-tunnel: w89 -> [_ w137]
                disable-tunnel: [_ w136] -> w88
                frame Enabled {
                  w93 = TRUE ("PAUSE")
                  n60 = call "ELAPSED TIMER VI FOR ramp speed.vi"("RESET"=w93, "PAUSE"=w93) -> ("error out"=w92:errorcluster)  [unwired: 7 in, 2 out]
                  n61 = while {
                    tunnel: w92 -> [_]
                    tunnel: w91 -> [w94]
                    stop <- w111 stop-if-true
                    w134 = FALSE ("PAUSE")
                    n62 = Unbundle By Name(w94) -> ("Main Screen.Test Duration"=w126:refnum<vi>)
                    n63 = Wait (ms)(milliseconds to wait=u32 10) -> ()  [unwired: 1 out]
                    n64 = property class="DigNum (strict)"(reference=w126) -> (reference out=w128:refnum<vi>, error out=w127:errorcluster, "Value"=w125:dbl)  [unwired: 1 in]
                    n65 = Unbundle By Name(w94) -> ("Main Screen.Start Test Temp"=w118:refnum<vi>)
                    n66 = Unbundle By Name(w94) -> ("Main Screen.STOP"=w121:refnum<vi>)
                    n67 = Close Reference(reference=w128, error in (no error)=w127) -> ()  [unwired: 1 out]
                    n68 = property class="Bool (strict)"(reference=w118) -> (reference out=w116:refnum<vi>, error out=w117:errorcluster, "Value"=w119:bool)  [unwired: 1 in]
                    n69 = property class="Bool (strict)"(reference=w121) -> (reference out=w123:refnum<vi>, error out=w122:errorcluster, "Value"=w120:bool)  [unwired: 1 in]
                    n70 = call "ELAPSED TIMER VI FOR ramp speed.vi"("TARGET"=w125, "RESET"=w134, "PAUSE"=w134) -> ("ELAPSED INDICATION"=w135:bool, "ELAPSED TIMER"=w132:dbl)  [unwired: 6 in, 1 out]
                    n71 = local read "Ramp Pattern"() -> (w129:dbl[])
                    n72 = Close Reference(reference=w116, error in (no error)=w117) -> ()  [unwired: 1 out]
                    n73 = Close Reference(reference=w123, error in (no error)=w122) -> ()  [unwired: 1 out]
                    n74 = Unbundle By Name(w94) -> ("SWAY.Mode Command"=w101:refnum<vi>)
                    n75 = Equal?(x=w119, y=FALSE) -> (x = y?=w114:bool)
                    n76 = Unbundle By Name(w94) -> ("SWAY.Distance"=w106:refnum<vi>)
                    n77 = Equal?(x=w120, y=TRUE) -> (x = y?=w115:bool)
                    n78 = And(x=w115, y=w114) -> (x .and. y?=w110:bool)
                    n79 = Array Size(array=w129) -> (size(s)=w133:i32)
                    n80 = Divide(x=w132, y=w125) -> (x/y=w131:dbl)
                    n81 = Unbundle By Name(w94) -> ("Main Screen.Set Speed"=w109:refnum<vi>)
                    n82 = Multiply(x=w133, y=w131) -> (x*y=w130:dbl)
                    n83 = property class="DigNum (strict)"(reference=w101, "Value"=u8 4) -> (reference out=w103:refnum<vi>, error out=w102:errorcluster)  [unwired: 1 in]
                    n84 = Index Array(array=w129, index=w130) -> (element=w95:dbl)
                    "Speed" <- w95
                    n85 = property class="DigNum (strict)"(reference=w106, "Value"=w95) -> (reference out=w104:refnum<vi>, error out=w105:errorcluster)  [unwired: 1 in]
                    n86 = Or(x=w110, y=w135) -> (x .or. y?=w111:bool)
                    n87 = property class="DigNum (strict)"(reference=w109, "Value"=w95) -> (reference out=w107:refnum<vi>, error out=w108:errorcluster)  [unwired: 1 in]
                    n88 = Close Reference(reference=w104, error in (no error)=w105) -> (error out=w98:errorcluster)
                    n89 = Close Reference(reference=w103, error in (no error)=w102) -> (error out=w99:errorcluster)
                    n90 = Merge Errors(w98, w99) -> (w97:errorcluster)
                    n91 = Close Reference(reference=w107, error in (no error)=w108) -> ()  [unwired: 1 out]
                    n92 = call "SWAY WRITE FGV.vi"("Enum - Menu"=Sway_Write_enum."WRITE", "error in (no error)"=w97, "main ref"=w94) -> ()  [unwired: 8 in, 1 out]
                  }
                }
                frame Disabled {
                  n93 = local read "Total Steps"() -> (w139:dbl)
                  n94 = for {
                    N: w139 -> [_]
                    tunnel: w138 -> [w140]
                    tunnel: w137 -> [w143]
                    tunnel: [w141] -> w136 mode=indexing
                    i -> [w164]
                    n95 = Unbundle By Name(w140) -> ("Motion Module.Motion Direction:  3"=w163:refnum<vi>)
                    n96 = Unbundle By Name(w140) -> ("SWAY.Mode Command"=w149:refnum<vi>)
                    n97 = Unbundle By Name(w140) -> ("Motion Module.Ramp Up 2"=w158:refnum<vi>)
                    n98 = property class="Ring (strict)"(reference=w163) -> (reference out=w161:refnum<vi>, error out=w162:errorcluster, "Value"=w160:u16)  [unwired: 1 in]
                    n99 = property class="Bool (strict)"(reference=w158) -> (reference out=w157:refnum<vi>, error out=w156:errorcluster, "Value"=w155:bool)  [unwired: 1 in]
                    n100 = property class="DigNum (strict)"(reference=w149, error in=w143, "Value"=u8 4) -> (reference out=w151:refnum<vi>, error out=w150:errorcluster)
                    n101 = local read "Wait Time"() -> (w165:dbl)
                    n102 = Close Reference(reference=w161, error in (no error)=w162) -> ()  [unwired: 1 out]
                    n103 = Wait (ms)(milliseconds to wait=w165) -> ()  [unwired: 1 out]
                    n104 = Close Reference(reference=w157, error in (no error)=w156) -> ()  [unwired: 1 out]
                    n105 = case shown="True" w155 {
                      tunnel: w164 -> [w167 w170]
                      tunnel: [w166 w169] -> w159
                      frame True {
                        n106 = local read "Initial Rpm"() -> (w168:dbl)
                        n107 = Add(x=w168, y=w167) -> (x+y=w166:dbl)
                      }
                      frame False {
                        n108 = local read "Initial Rpm"() -> (w171:dbl)
                        n109 = Subtract(x=w171, y=w170) -> (x-y=w169:dbl)
                      }
                    }
                    n110 = Close Reference(reference=w151, error in (no error)=w150) -> (error out=w147:errorcluster)
                    n111 = Unbundle By Name(w140) -> ("SWAY.Distance"=w154:refnum<vi>)
                    n112 = case shown="1" w160 {
                      tunnel: [w172 w174] -> w142
                      tunnel: w159 -> [w172 w173]
                      frame 0, Default {
                      }
                      frame 1 {
                        n113 = Negate(x=w173) -> (-x=w174:dbl)
                      }
                    }
                    n114 = property class="DigNum (strict)"(reference=w154, "Value"=w142) -> (reference out=w152:refnum<vi>, error out=w153:errorcluster)  [unwired: 1 in]
                    n115 = Close Reference(reference=w152, error in (no error)=w153) -> (error out=w146:errorcluster)
                    n116 = Merge Errors(w146, w147) -> (w145:errorcluster)
                    n117 = call "SWAY WRITE FGV.vi"("Enum - Menu"=Sway_Write_enum."WRITE", "error in (no error)"=w145, "main ref"=w140) -> ("error out"=w141:errorcluster)  [unwired: 8 in]
                  }
                }
              }
            }
            frame #2 {
              n118 = disable-structure shown="Enabled" {
                disable-tunnel: w176 -> [w198 w201]
                disable-tunnel: [w196 w201] -> _
                disable-tunnel: w175 -> [w195 _]
                frame Disabled {
                  n119 = call "PID UNLOAD.vi"("error in (no error)"=w198, "main ref"=w195) -> ("error out"=w200:errorcluster)  [unwired: 9 in]
                  n120 = call "HEAVE WRITE FGV.vi"("Enum - Menu"=Heave_Write_enum."WRITE", "error in (no error)"=w200, "main ref"=w195) -> ("error out"=w197:errorcluster)  [unwired: 8 in]
                  n121 = call "SWAY UNIFORM SPEED STOP.vi"("error in (no error)"=w197, "Data Cluster"=w195) -> ("error out"=w196:errorcluster)  [unwired: 9 in]
                }
                frame Enabled {
                }
              }
              n122 = Unbundle By Name(w175) -> ("Main Screen.Start Test"=w190:refnum<vi>)
              n123 = Unbundle By Name(w175) -> ("Main Screen.STOP"=w179:refnum<vi>)
              n124 = Unbundle By Name(w175) -> ("Main Screen.Start Test Temp"=w180:refnum<vi>)
              n125 = Unbundle By Name(w175) -> ("Main Screen.Load En"=w188:refnum<vi>)
              n126 = property class="Bool (strict)"(reference=w179, "Value"=FALSE, "Visible"=TRUE) -> (reference out=w177:refnum<vi>, error out=w178:errorcluster)  [unwired: 1 in]
              n127 = property class="Bool (strict)"(reference=w180, "Value"=FALSE) -> (reference out=w182:refnum<vi>, error out=w181:errorcluster)  [unwired: 1 in]
              n128 = property class="Bool (strict)"(reference=w188, "Value"=FALSE) -> (reference out=w186:refnum<vi>, error out=w187:errorcluster)  [unwired: 1 in]
              n129 = property class="Bool (strict)"(reference=w190, "Value"=FALSE, "Visible"=TRUE) -> (reference out=w192:refnum<vi>, error out=w191:errorcluster)  [unwired: 1 in]
              n130 = Close Reference(reference=w177, error in (no error)=w178) -> ()  [unwired: 1 out]
              n131 = Close Reference(reference=w182, error in (no error)=w181) -> ()  [unwired: 1 out]
              n132 = Close Reference(reference=w186, error in (no error)=w187) -> ()  [unwired: 1 out]
              n133 = Close Reference(reference=w192, error in (no error)=w191) -> ()  [unwired: 1 out]
            }
          }
        }
      }
    }
    frame Error {
    }
  }
